vi "Parse Core.vi"(0 "SA Path in":refnum<class "SA Path.lvclass">, 5 "Config Row":string[](array[string]), 11 "error in":errorcluster) -> (4 "SA Path out":refnum<class "SA Path.lvclass">, 15 "error out":errorcluster)   [LabVIEW 2023, in "RFFixtureCharact.Public.lvlib" / "SA Path.lvclass"]
uses:
  SA Path.lvclass
  C:/srd-semi-rfcal-software/AuxTools/STSRFFixtureCharactUtility/Source/Code Modules/Common/Base Classes/Path/Path.lvclass
  Common/Base Classes/Path/Path.lvclass/Path.ctl
  Common/Base Classes/Path/Properties/Read Interval.vi
  SA Path.lvclass/SA Path.ctl
  SA Abstract Path/SA Abstract Path.lvclass
  Common/RFCalAndFixtureCharact.Common.lvlib
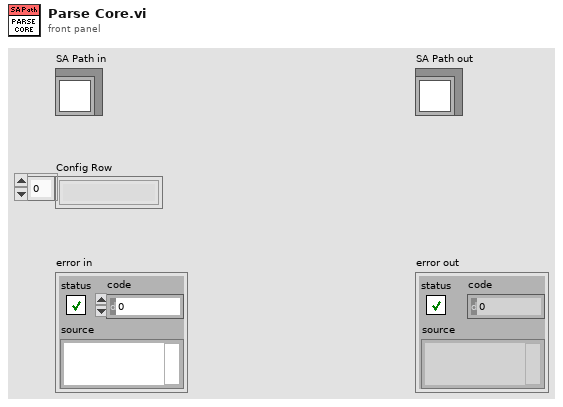
[diagram p1: front panel]
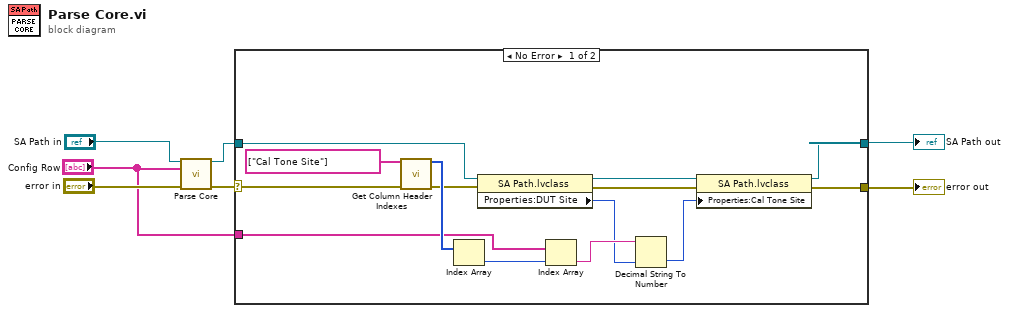
[diagram p0: block diagram]
diagram:
  n1 = call-parent "Parse Core.vi"("SA Path in"="SA Path in", "Config Row"="Config Row", "error in (no error)"="error in") -> ("SA Path out"=w6:refnum<class "SA Path.lvclass">, "error out"=w5:errorcluster)  [unwired: 11 in]
  n2 = case shown="No Error" w5 {
    selector: w5 -> [w16 w23]
    tunnel: w6 -> [w15 w22]
    tunnel: [w21 w23] -> w4
    tunnel: [w8 w22] -> w3
    tunnel: "Config Row" -> [w12 _]
    frame No Error {
      n3 = call "Get Column Header Indexes.vi"("Column Header Names"=string[] ["Cal Tone Site"], "error in"=w16) -> ("Column Header Indices"=w19:i32[], "error out"=w14:errorcluster)  [unwired: 11 in, 1 out]
      n4 = Index Array(array=w19) -> (element=w18:i32)  [unwired: 1 in]
      n5 = property class="SA Path.lvclass"(reference=w15, error in=w14) -> (reference out=w17:refnum<class "SA Path.lvclass">, error out=w9:errorcluster, "Properties:DUT Site"=w11:i32)
      n6 = Index Array(array=w12, index=w18) -> (element=w13:string)
      n7 = Decimal String To Number(string=w13, default (0L)=w11) -> (number=w10:i32)  [unwired: 1 in, 1 out]
      n8 = property class="SA Path.lvclass"(reference=w17, error in=w9, "Properties:Cal Tone Site"=w10) -> (reference out=w8:refnum<class "SA Path.lvclass">, error out=w21:errorcluster)
    }
    frame Error {
    }
  }
  "error out" <- w4
  "SA Path out" <- w3
